vi "subvi_Get_data.vi"(8 "에러 입력(에러 없음)":errorcluster, 11 "Modbus Master 입력":refnum<class "Modbus Master.lvclass">) -> (0 "에러 출력":errorcluster, 2 "register values":u16[](array[numeric]), 3 "Modbus Master 출력":refnum<class "Modbus Master.lvclass">)   [LabVIEW 2016]
uses:
  <vilib>/NI/Modbus Library/API/Master/Modbus Master.lvclass
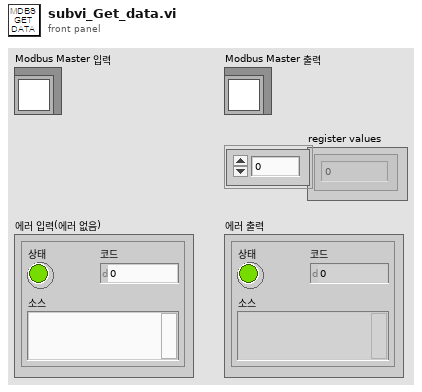
[diagram p1: front panel]
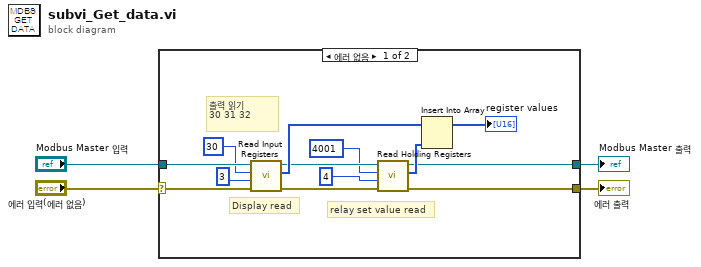
[diagram p0: block diagram]
diagram:
  n1 = case shown="에러 없음" "에러 입력(에러 없음)" {
    selector: "에러 입력(에러 없음)" -> [w13 w19]
    tunnel: "Modbus Master 입력" -> [w14 w18]
    tunnel: [w12 w19] -> w2
    tunnel: [w11 w18] -> w1
    frame No Error {
      # "relay set value read"
      # "출력 읽기\n30 31 32"
      # "Display read"
      n2 = call-dynamic "Read Input Registers.vi"("error in"=w13, "number of inputs"=u16 3, "starting address"=u16 30, "Modbus master in"=w14) -> ("error out"=w10:errorcluster, "register values"=w16:u16[], "Modbus master out"=w9:refnum<class "Modbus Master.lvclass">)  [unwired: 5 in]
      n3 = call-dynamic "Read Holding Registers.vi"("error in"=w10, "number of inputs"=u16 4, "starting address"=u16 4001, "Modbus master in"=w9) -> ("error out"=w12:errorcluster, "register values"=w15:u16[], "Modbus master out"=w11:refnum<class "Modbus Master.lvclass">)  [unwired: 5 in]
      n4 = Insert Into Array(array=w16, new element=w15) -> (→"register values":u16[])  [unwired: 1 in]
    }
    frame Error {
    }
  }
  "에러 출력" <- w2
  "Modbus Master 출력" <- w1
